vi "prelim_toggle_general_ctrls.vi"(8 "error in":errorcluster, 11 "reference cluster":T1) -> (0 "error out":errorcluster, 3 "reference cluster":T1)   [LabVIEW 2016]
uses:
  Type Definitions/reference_cluster.ctl
  Type Definitions/vars_settings.ctl
  Type Definitions/stim_type.ctl
  Type Definitions/backlight_type.ctl
  Type Definitions/vars_runtime.ctl
  Type Definitions/data.ctl
  Type Definitions/notifier_elements_GUI.ctl
  Type Definitions/notifier_elements_DAQ.ctl
  Type Definitions/notifier_elements_write.ctl
  Type Definitions/control_references.ctl
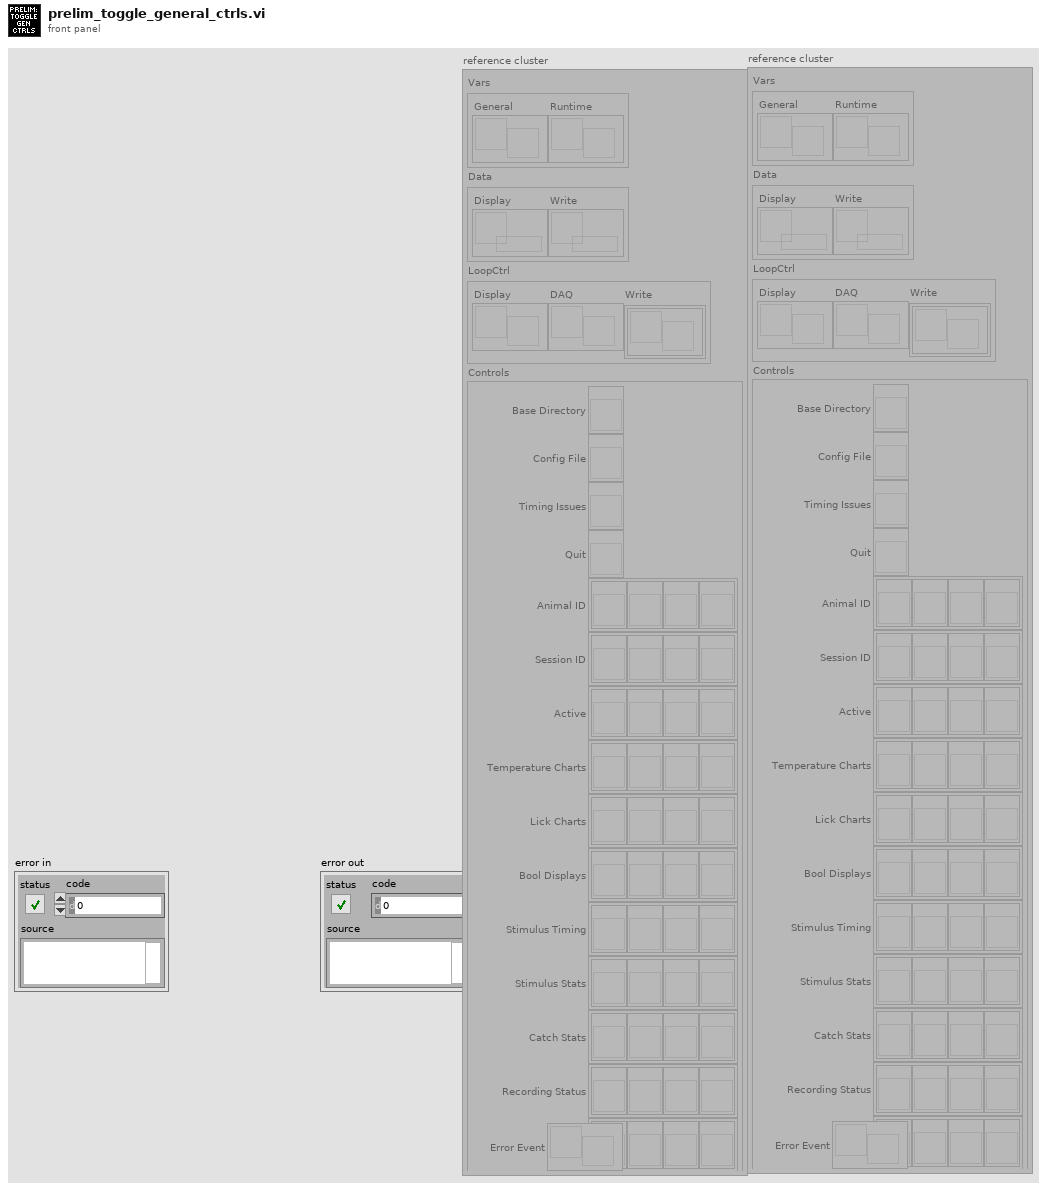
[diagram p1: front panel]
types:
  T1 = typedef "reference_cluster.ctl" = cluster{"Vars":cluster{"General":refnum<notifier>, "Runtime":refnum<notifier>}, "Data":cluster{"Display":refnum<queue>, "Write":refnum<queue>}, "LoopCtrl":cluster{"Display":refnum<notifier>, "DAQ":refnum<notifier>, "Write":refnum<notifier>[]}, "Controls":T2, "Error Event":refnum<user-event>}
  T2 = typedef "control_references.ctl" = cluster{"Base Directory":refnum<vi>, "Config File":refnum<vi>, "Timing Issues":refnum<vi>, "Quit":refnum<vi>, "Animal ID":refnum<vi>[], "Session ID":refnum<vi>[], "Active":refnum<vi>[], "Temperature Charts":refnum<vi>[], "Lick Charts":refnum<vi>[], "Bool Displays":refnum<vi>[], "Stimulus Timing":refnum<vi>[], "Stimulus Stats":refnum<vi>[], "Catch Stats":refnum<vi>[], "Recording Status":refnum<vi>[], "Pairing":refnum<vi>[]}
  T3 = enum8{"Enabled", "Disabled", "Disabled and Grayed Out"}
  T4 = enum8{"Enabled", "Disabled", "Disabled and Grayed Out"}[]
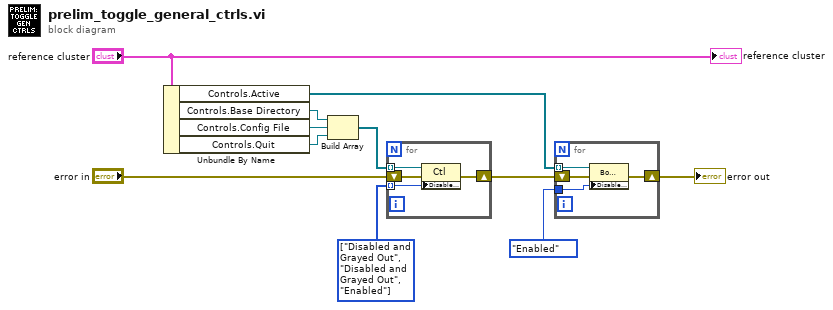
[diagram p0: block diagram]
diagram:
  w10 = T4 [enum."Disabled and Grayed Out", enum."Disabled and Grayed Out", enum."Enabled"] items=["Enabled", "Disabled", "Disabled and Grayed Out"] ("Disabled")
  n1 = Unbundle By Name("reference cluster") -> ("Controls.Active"=w4:refnum<vi>[], "Controls.Base Directory"=w7:refnum<vi>, "Controls.Config File"=w6:refnum<vi>, "Controls.Quit"=w5:refnum<vi>)
  n2 = Build Array(w7, w6, w5) -> (w9:refnum<vi>[])
  n3 = for {
    tunnel: w9 -> [w15] mode=indexing
    tunnel: w10 -> [w14] mode=indexing
    shift-right: [w12] -> w2
    shift-left: "error in" -> [w13]
    n4 = property class="Ctl"(reference=w15, error in=w13, "DisabledEnum"=w14) -> (error out=w12:errorcluster)  [unwired: 1 out]
  }
  n5 = for {
    tunnel: w4 -> [w19] mode=indexing
    tunnel: T3."Enabled" ("Disabled") -> [w18]
    shift-right: [w16] -> w1
    shift-left: w2 -> [w17]
    n6 = property class="Bool (strict)"(reference=w19, error in=w17, "DisabledEnum"=w18) -> (error out=w16:errorcluster)  [unwired: 1 out]
  }
  "error out" <- w1
  "reference cluster" <- "reference cluster"
